vi "Word Game.vi"() -> ()   [LabVIEW 2015]
uses:
  TypeDef/Word.ctl
panel:
  in  "Check":bool
  in  "Word 6":T1
  in  "Word 5":T1
  in  "Word 4":T1
  in  "Word 3":T1
  in  "Word 2":T1
  in  "Word 1":T1
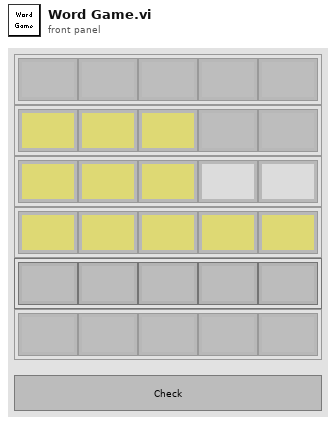
[diagram p1: front panel]
types:
  T1 = typedef "Word.ctl" = cluster{"1":string, "2":string, "3":string, "4":string, "5":string}
  T2 = enum8{"Enabled", "Disabled", "Disabled and Grayed Out"}
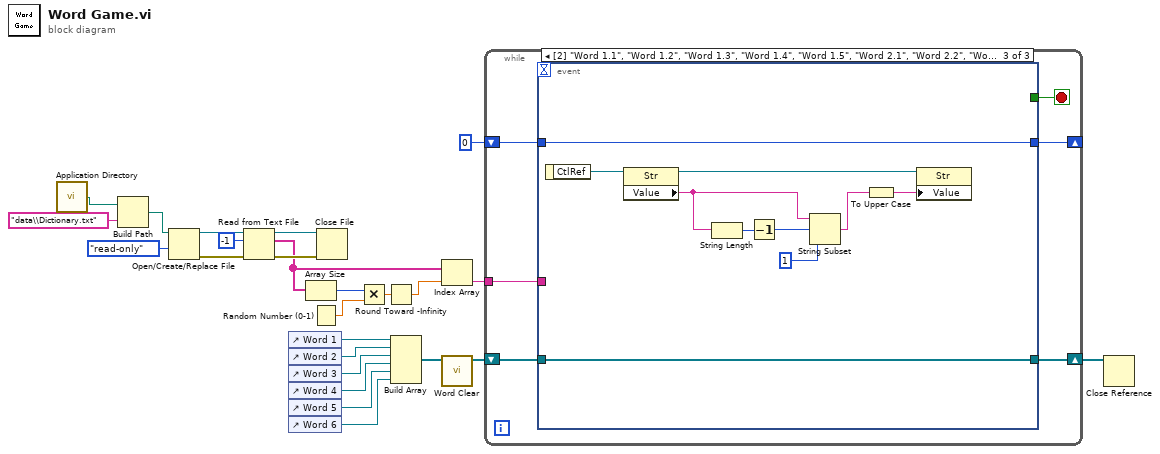
[diagram p0: block diagram]
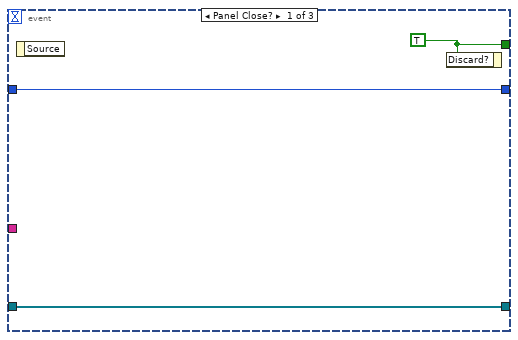
[diagram p2: hidden frame]
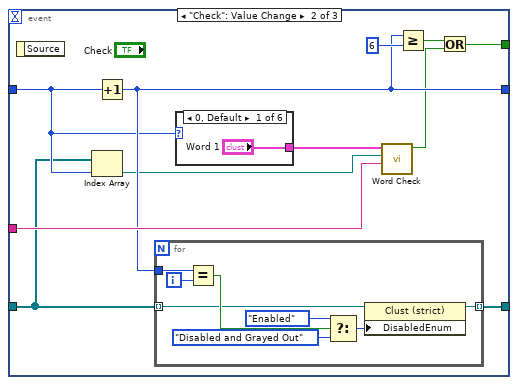
[diagram p3: hidden frame]
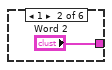
[diagram p4: hidden frame]
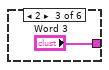
[diagram p5: hidden frame]
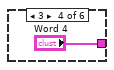
[diagram p6: hidden frame]
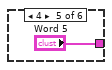
[diagram p7: hidden frame]
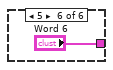
[diagram p8: hidden frame]
diagram:
  n1 = call <vilib>:"Application Directory.vi"() -> ("Application Directory"=w17:path)
  n2 = Build Path(base path=w17, name or relative path="data\\Dictionary.txt") -> (appended path=w19:path)
  n3 = Open/Create/Replace File(file path (use dialog)=w19, access (0:read/write)=enum16{"read/write", "read-only", "write-only"}."read-only") -> (refnum out=w24:refnum<file>, error out=w23:errorcluster)  [unwired: 4 in, 1 out]
  n4 = Read from Text File(file (use dialog)=w24, count=-1, error in=w23) -> (refnum out=w21:refnum<file>, text=w13:string[], error out=w20:errorcluster)  [unwired: 1 in, 1 out]
  n5 = control-ref of="Word 1"() -> (w9:refnum<vi>)
  n6 = control-ref of="Word 2"() -> (w8:refnum<vi>)
  n7 = control-ref of="Word 3"() -> (w7:refnum<vi>)
  n8 = control-ref of="Word 4"() -> (w6:refnum<vi>)
  n9 = control-ref of="Word 5"() -> (w5:refnum<vi>)
  n10 = control-ref of="Word 6"() -> (w4:refnum<vi>)
  n11 = Array Size(array=w13) -> (size(s)=w16:i32)
  n12 = Random Number (0-1)() -> (number: 0 to 1=w15:dbl)
  n13 = Close File(refnum=w21, error in=w20) -> ()  [unwired: 2 out]
  n14 = Multiply(x=w16, y=w15) -> (x*y=w14:dbl)
  n15 = Round Toward -Infinity(1:w14) -> (0:w12:dbl)
  n16 = Build Array(w9, w8, w7, w6, w5, w4) -> (w3:refnum<vi>[])
  n17 = Index Array(array=w13, index=w12) -> (element=w11:string)
  n18 = call "Word Clear.vi"("Words_Ref in"=w3) -> ("Words_Ref out"=w2:refnum<vi>[])  [unwired: 10 in]
  n19 = while {
    tunnel: w11 -> [w30]
    shift-right: [w28] -> _
    shift-left: 0 -> [w29]
    shift-right: [w26] -> w1
    shift-left: w2 -> [w27]
    stop <- w31 stop-if-true
    n20 = event shown="[2] \"Word 1.1\", \"Word 1.2\", \"Word 1.3\", \"Word 1.4\", \"Word 1.5\", \"Word 2.1\", \"Word 2.2\", \"Word 2.3\", \"Word 2.4\", \"Word 2.5\", \"Word 3.1\", \"Word 3.2\", \"Word 3.3\", \"Word 3.4\", \"Word 3.5\", \"Word 4.1\", \"Word 4.2\", \"Word 4.3\", \"Word 4.4\", \"Word 4.5\", \"Word 5.1\", \"Word 5.2\", \"Word 5.3\", \"Word 5.4\", \"Word 5.5\", \"Word 6.1\", \"Word 6.2\", \"Word 6.3\", \"Word 6.4\", \"Word 6.5\": Value Change" {
      selector: _ -> [_ _ _]
      dyn-events: _ -> [_ _ _]
      timeout: _ -> [_ _ _]
      tunnel: [w34 w41 _] -> w31
      tunnel: w30 -> [_ w43 _]
      tunnel: w29 -> [w33 w37 w69]
      tunnel: [w33 w42 w69] -> w28
      tunnel: w27 -> [w32 w36 w60]
      tunnel: [w32 w38 w60] -> w26
      event Panel Close? {
        w34 = TRUE
        n21 = event-data() -> ()  [unwired: 1 in, 1 out]
        n22 = event-data("Discard?"=w34) -> ()  [unwired: 1 in, 1 out]
      }
      event "Check": Value Change {
        n23 = event-data() -> ()  [unwired: 1 in, 1 out]
        n24 = Index Array(array=w36, index=w37) -> (element=w35:refnum<vi>)
        n25 = Increment(x=w37) -> (x+1=w42:i32)
        n26 = for {
          tunnel: w36 -> [w47] mode=indexing
          tunnel: w42 -> [w53]
          tunnel: [w46] -> w38 mode=indexing
          i -> [w52]
          n27 = Equal?(x=w53, y=w52) -> (x = y?=w48:bool)
          n28 = Select(t=T2."Enabled" ("Disabled"), s=w48, f=T2."Disabled and Grayed Out" ("Disabled")) -> (s? t:f=w49:T2)
          n29 = property class="Clust (strict)"(reference=w47, "DisabledEnum"=w49) -> (reference out=w46:refnum<vi>)  [unwired: 1 in, 1 out]
        }
        n30 = case shown="0, Default" w37 {
          tunnel: ["Word 1" "Word 2" "Word 3" "Word 4" "Word 5" "Word 6"] -> w44
          frame 0, Default {
          }
          frame 1 {
          }
          frame 2 {
          }
          frame 3 {
          }
          frame 4 {
          }
          frame 5 {
          }
        }
        n31 = call "Word Check.vi"("Any"=w43, "Word_Ref"=w35, "Word"=w44) -> ("IsOk"=w39:bool)  [unwired: 8 in]
        n32 = Greater Or Equal?(x=w42, y=6) -> (x >= y?=w40:bool)
        n33 = Or(x=w40, y=w39) -> (x .or. y?=w41:bool)
      }
      event Value Change {
        n34 = event-data() -> ("CtlRef"=w68:refnum<vi>)  [unwired: 1 in]
        n35 = property class="Str"(reference=w68) -> (reference out=w67:refnum<vi>, "Value"=w62:string)  [unwired: 1 in, 1 out]
        n36 = String Length(string=w62) -> (length=w66:i32)
        n37 = Decrement(x=w66) -> (x-1=w65:i32)
        n38 = String Subset(string=w62, offset (0)=w65, length (rest)=1 ("length (rest)")) -> (substring=w63:string)
        n39 = To Upper Case(1:w63) -> (0:w61:string)
        n40 = property class="Str"(reference=w67, "Value"=w61) -> ()  [unwired: 1 in, 2 out]
      }
    }
  }
  n41 = Close Reference(reference=w1) -> ()  [unwired: 1 in, 1 out]
